vi "New Password.vi"(8 "Error in":errorcluster, 11 "Username":string) -> (0 "Error out":errorcluster)   [LabVIEW 2019, in "User Lib.lvlib"]
uses:
  User Lib.lvlib
  <vilib>/addons/database/Connection.llb/DB Tools Open Connec (String).vi
  <vilib>/addons/database/_DB Variant To Data/Database Variant To Data.xnode
  <vilib>/addons/database/NI_Database_API.lvlib
  database.lvlib
panel:
  in  "Cancel":bool
  in  "OK":bool
  in  "Old Password":string
  in  "Confirm New Password":string
  in  "New Password":string
  out "Username 2":string caption="Username"
  # "New Password"
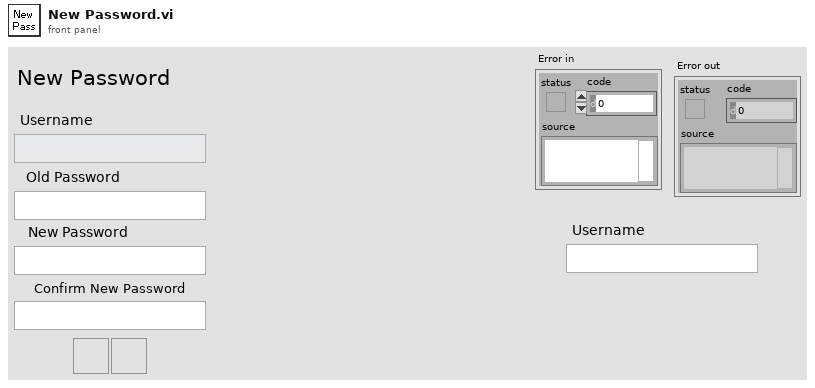
[diagram p1: front panel]
types:
  T1 = typedef "NI_Database_API.lvlib/Conn ObjectReference.ctl" = refnum<k1>
  T2 = cluster{i32, "date/time string":string, "date/time string":string, string}
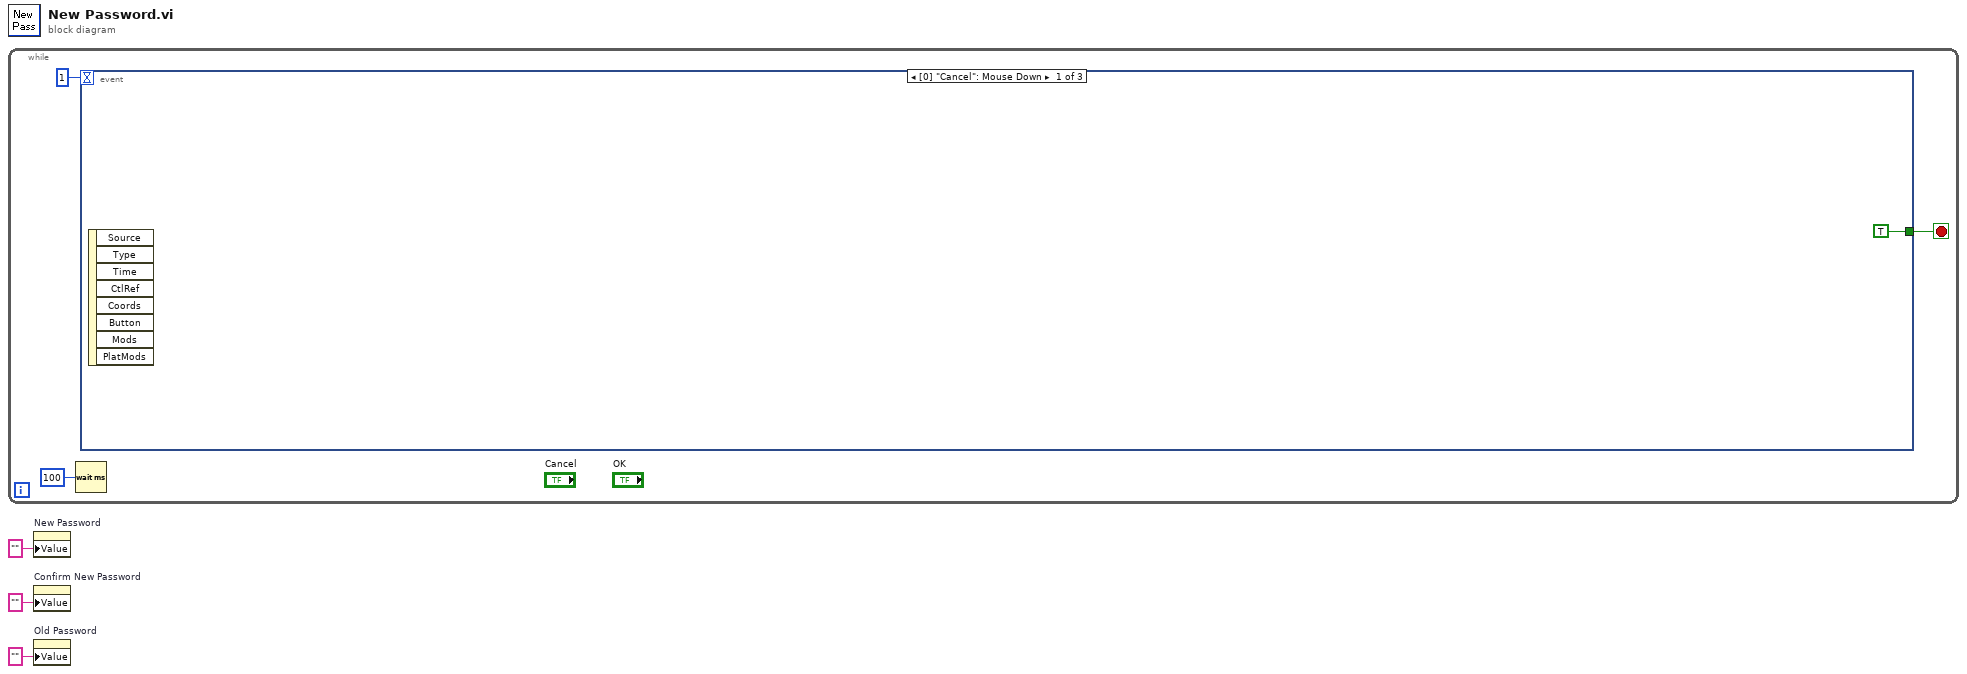
[diagram p0: block diagram]
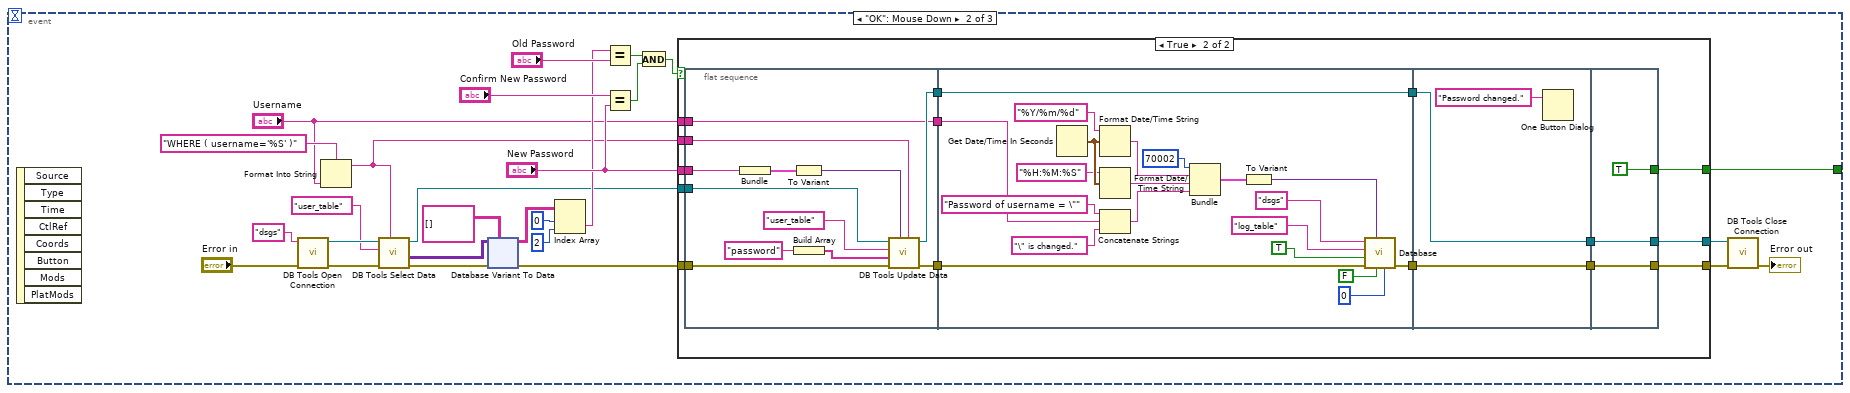
[diagram p2: hidden frame]
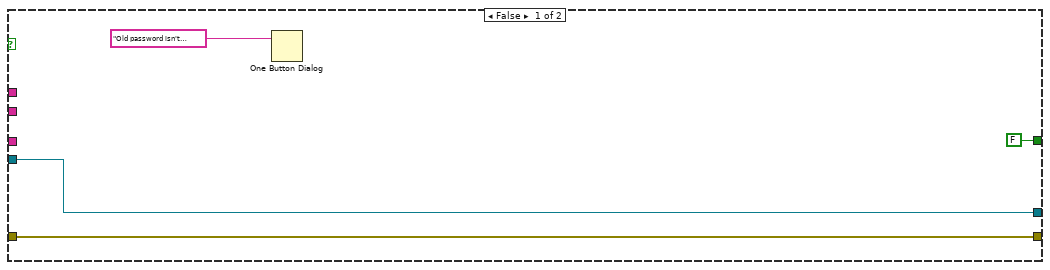
[diagram p3: hidden frame]
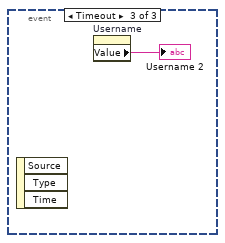
[diagram p4: hidden frame]
diagram:
  n1 = while {
    stop <- w5 stop-if-true
    n2 = Wait (ms)(milliseconds to wait=u32 100) -> ()  [unwired: 1 out]
    n3 = event shown="[0] \"Cancel\": Mouse Down" {
      selector: _ -> [_ _ _]
      dyn-events: _ -> [_ _ _]
      timeout: 1 -> [_ _ _]
      tunnel: [TRUE w9 _] -> w5
      event "Cancel": Mouse Down {
        n4 = event-data() -> ()  [unwired: 1 in, 8 out]
      }
      event "OK": Mouse Down {
        n5 = event-data() -> ()  [unwired: 1 in, 8 out]
        n6 = call-poly <vilib>:"DB Tools Open Connection.vi"("error in (no error)"="Error in", "connection information"="dsgs") -> ("error out"=w16:errorcluster, "connection reference"=w17:T1)  [unwired: 6 in]
        n7 = Format Into String(format string="WHERE ( username='%S' )" ("condition"), "Username") -> (resulting string=w21:string)  [unwired: 2 in, 1 out]
        n8 = call <vilib>:"DB Tools Select Data.vi"("condition"=w21, "error in (no error)"=w16, "table"="user_table", "connection reference"=w17) -> ("error out"=w23:errorcluster, "data"=w22:variant[][], "connection reference out"=w18:T1)  [unwired: 2 in]
        n9 = xnode "Database Variant To Data"("database variant"=w22, "error in (no error)"=w23, "type"=string[][] []) -> ("data"=w25:string[][], "error out"=w24:errorcluster)
        n10 = Index Array(array=w25, index (row)=0 ("disabled index (row)"), index (col)=2 ("disabled index (col)")) -> (element=w26:string)
        n11 = Equal?(x=w26, y="Old Password") -> (x = y?=w27:bool)
        n12 = Equal?(x="Confirm New Password", y="New Password") -> (x = y?=w28:bool)
        n13 = And(x=w27, y=w28) -> (x .and. y?=w29:bool)
        n14 = case shown="True" w29 {
          tunnel: w21 -> [_ w97]
          tunnel: "New Password" -> [_ w96]
          tunnel: w24 -> [w81 w94]
          tunnel: w18 -> [w82 w95]
          tunnel: [w81 w93] -> w19
          tunnel: [w82 w92] -> w20
          tunnel: [FALSE w85] -> w9
          tunnel: "Username" -> [_ w83]
          frame False {
            n15 = One Button Dialog(message="Old password isn't correct or new password does not confirm.") -> ()  [unwired: 1 in, 1 out]
          }
          frame True {
            n16 = flat-sequence {
              tunnel: w97 -> [w107]
              tunnel: w96 -> [w105]
              tunnel: w95 -> [w102]
              tunnel: w94 -> [w101]
              tunnel: [w100] -> w91
              tunnel: [w99] -> w90
              tunnel: [w98] -> w84
              tunnel: w83 -> [w98]
              tunnel: w91 -> [w115]
              tunnel: w90 -> [w129]
              tunnel: [w114] -> w89
              tunnel: [w129] -> w88
              tunnel: w84 -> [w112]
              tunnel: w89 -> [w132]
              tunnel: w88 -> [w131]
              tunnel: [w132] -> w87
              tunnel: [w131] -> w86
              tunnel: [w134] -> w92
              tunnel: [w135] -> w93
              tunnel: w87 -> [w135]
              tunnel: w86 -> [w134]
              tunnel: [TRUE] -> w85
              frame #0 {
                n17 = Bundle("New Password"=w105) -> (w104:cluster{"New Password":string})  [unwired: 1 in]
                n18 = To Variant(anything=w104) -> (Variant=w103:variant)
                n19 = Build Array("password" ("table")) -> (w109:string[])
                n20 = call <vilib>:"DB Tools Update Data.vi"("condition"=w107, "data"=w103, "error in (no error)"=w101, "columns"=w109, "table"="user_table", "connection reference"=w102) -> ("error out"=w100:errorcluster, "connection reference out"=w99:T1)  [unwired: 4 in]
              }
              frame #1 {
                n21 = Get Date/Time In Seconds() -> (seconds since 1Jan1904=w124:timestamp)
                n22 = Format Date/Time String(time format string (%c)="%Y/%m/%d", seconds (now)=w124) -> (date/time string=w125:string)  [unwired: 1 in]
                n23 = Format Date/Time String(time format string (%c)="%H:%M:%S", seconds (now)=w124) -> (date/time string=w126:string)  [unwired: 1 in]
                n24 = Concatenate Strings("Password of username = \"" ("string"), w112, "\" is changed." ("string")) -> (w111:string)
                n25 = Bundle(70002, "date/time string"=w125, "date/time string"=w126, w111) -> (w127:T2)  [unwired: 1 in]
                n26 = To Variant(anything=w127) -> (Variant=w128:variant)
                n27 = call "Database.vi"("Maximum Row"=u64 0 ("Storage Time (Day)"), "Delete row?"=FALSE, "Data"=w128, "Error in"=w115, "Auto Increment ID?"=TRUE, "Table"="log_table" ("table"), "Connection"="dsgs" ("table")) -> ("Error out"=w114:errorcluster)  [unwired: 4 in]
              }
              frame #2 {
                n28 = One Button Dialog(message="Password changed.") -> ()  [unwired: 1 in, 1 out]
              }
              frame #3 {
              }
            }
          }
        }
        n29 = call <vilib>:"DB Tools Close Connection.vi"("error in (no error)"=w19, "connection reference"=w20) -> ("error out"=→"Error out":errorcluster)  [unwired: 5 in]
      }
      event Timeout {
        n30 = event-data() -> ()  [unwired: 1 in, 3 out]
        n31 = property on="Username" class="Str"() -> ("Value"=→"Username 2":string)  [unwired: 2 in, 2 out]
      }
    }
  }
  n32 = property on="New Password" class="Str"("Value"="" ("New Password")) -> ()  [unwired: 2 in, 2 out]
  n33 = property on="Confirm New Password" class="Str"("Value"="" ("New Password")) -> ()  [unwired: 2 in, 2 out]
  n34 = property on="Old Password" class="Str"("Value"="" ("New Password")) -> ()  [unwired: 2 in, 2 out]
